vi "Simple ReaderWriteri.vi"() -> ()   [LabVIEW 2012]
uses:
  <vilib>/Platform/TimedLoop/XDataNode/timing_clust.ctl
  <vilib>/Platform/TimedLoop/XDataNode/nitl_modes.ctl
  <vilib>/Platform/TimedLoop/XDataNode/wakeup.ctl
  <vilib>/rvi/Emulation/niFpgaSctlEmulationRegisterWithScheduler.vi
  <vilib>/rvi/eio/common/nirviEmuTemplateMethod_errors.vi
  <vilib>/rvi/Emulation/niFpgaSctlEmulationScheduler.vi
  <vilib>/rvi/interface/RandomDataEmulation/nirviRandomDataFPGAFIFO.vi
  <vilib>/rvi/interface/RandomDataEmulation/niFpgaRandomDataHandleErrors.vi
  <vilib>/Platform/TimedLoop/XDataNode/XDataNode.xnode
  <vilib>/eio/EIONode/EIONode.xnode
  <vilib>/rvi/DataTransferAndStorage/Container/XNode/niFpgaContainer.xnode
  <vilib>/rvi/interface/RandomDataEmulation/nirviRandomDataFpgaReadWriteTemplate.vi
  <vilib>/Platform/TimedLoop/XDataNode/XDNodeRunTimeDep.lvlib
panel:
  out "All samples acquired":bool
  in  "Write array (Ch1)":bool[](array[boolean])=[FALSE, FALSE, FALSE, FALSE, FALSE, FALSE, FALSE, FALSE, FALSE, FALSE, FALSE, FALSE, FALSE, FALSE, FALSE, FALSE]
  in  "Samples":i32
  in  "Onboard_Clock_Write_Data":u16 format="%b"
  in  "Onboard_Clock_Write":bool
  out "Onboard_Clock_Ready":bool
  out "Read array (Ch0)":bool[](array[boolean])
  in  "Acq_Reset":bool
  in  "Clock Source":u8(ring)=3 items=["Tristate"=0, "Sync Clock (PXIe Only)"=2, "Adapter Module Onboard Clock"=3, "Strobe From Crosspoint Switch"=4, "Strobe Bypass"=5]
  in  "Xpoint_Switch_Write":bool
  out "Xpoint_Switch_Ready":bool
  in  "Commit":bool
  # "Configuration"
  # "Read on Ch0, Write on Ch1"
  # "Generation"
  # "Acquisition"
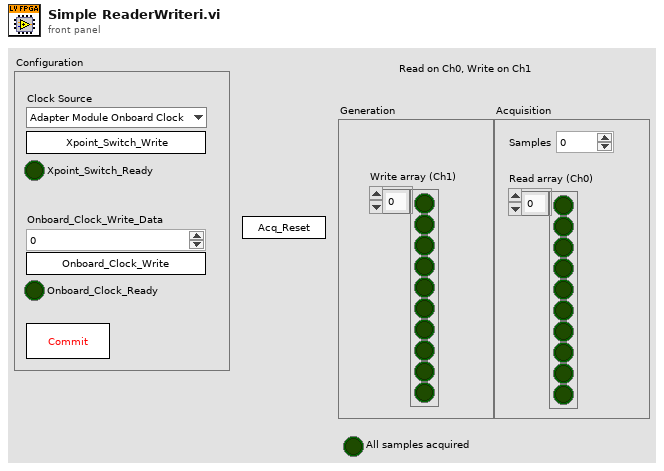
[diagram p1: front panel]
types:
  T1 = typedef "XDNodeRunTimeDep.lvlib/timing_clust.ctl" = cluster{"Expected End [f-1]":u64, "Actual End [f-1]":u64, "Finished Late? [f-1]":bool, "Expected End [i-1]":u64, "Actual End [i-1]":u64, "Finished Late? [i-1]":bool, "Expected Start [i]":u64, "Actual Start [i]":u64, "Expected Start [f]":u64, "Actual Start [f]":u64, "Source Name":string, "Structure Name":string, "Period":i64, "Deadline":i64, "Offset":i64, "Start":i64, "Priority":i32, "Timeout":i32, "Mode":T2, "Wakeup Reason":T3, "Error":errorcluster, "Source Type":string, "Secondary Source Type":string, "Global End Time":u64, "Global Start Time":u64, "Frame Duration":u64, "Iteration Duration":u64, "Assigned CPU":i32, "I/O Scan Engine Mode":u32}
  T2 = typedef "XDNodeRunTimeDep.lvlib/nitl_modes.ctl" = enum32{"No Change", "Process missed periods, maintain original phase", "Discard missed periods, maintain original phase", "Process missed periods, ignore original phase", "Discard missed periods, ignore original phase"}
  T3 = typedef "XDNodeRunTimeDep.lvlib/wakeup.ctl" = enum32{"Normal", "Aborted", "Asynchronous wakeup", "Timing source error", "Timed loop error", "Timeout"}
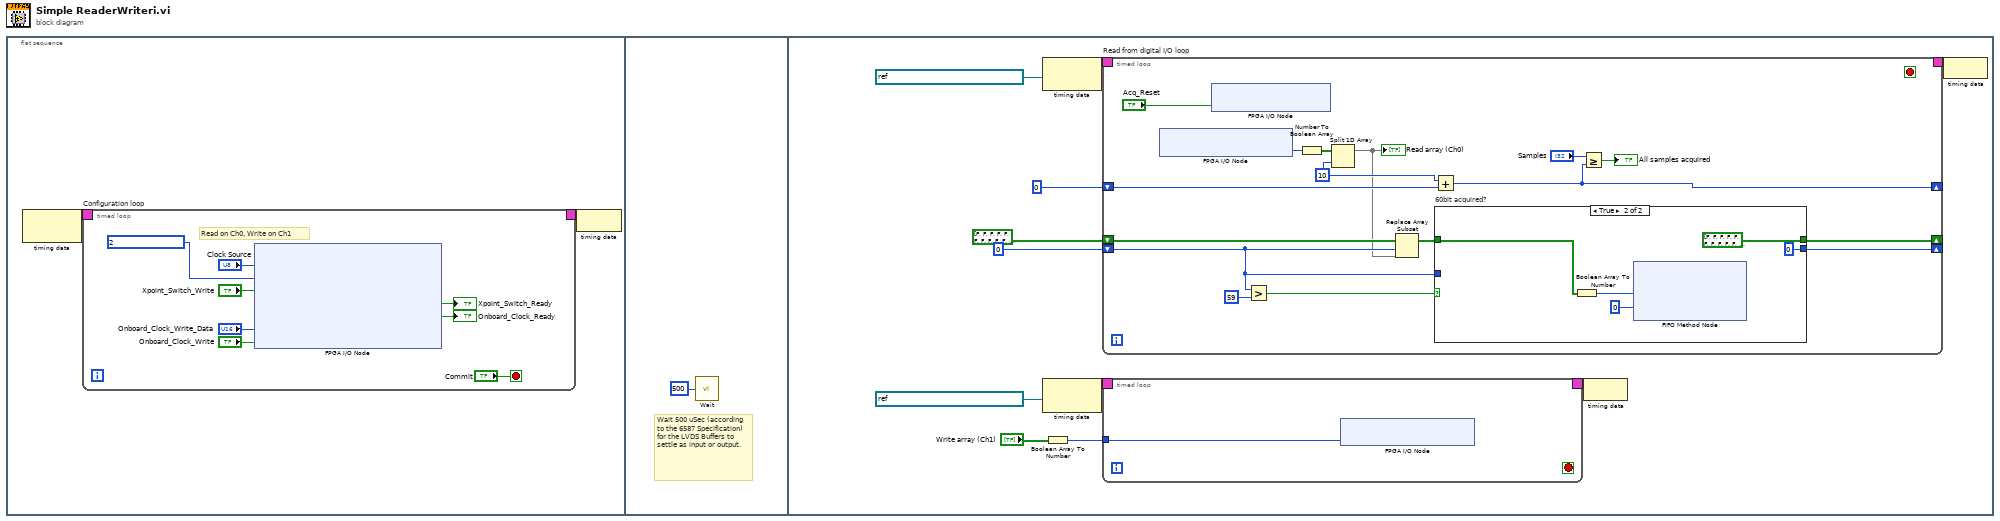
[diagram p0: block diagram]
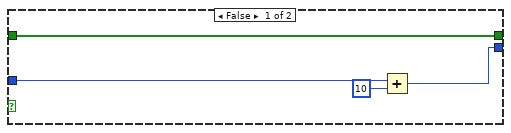
[diagram p2: hidden frame]
diagram:
  n1 = flat-sequence {
    frame #0 {
      n2 = node-c288() -> (w2:T1)  [unwired: 1 in]
      n3 = timed-loop "Configuration loop" {
        timing: w2 -> [_]
        timing-out: [_] -> w1
        stop <- "Commit" stop-if-true
        # "Read on Ch0, Write on Ch1"
        n4 = xnode "FPGA I/O Node"("IO Module\\Acq_IO_Clock_Source"="Clock Source", "IO Module\\LVDS_Data_Dir"=u16 2 ("IO Module\\LVDS_Data_Dir"), "IO Module\\Xpoint_Switch_Write"="Xpoint_Switch_Write", "IO Module\\Onboard_Clock_Write_Data"="Onboard_Clock_Write_Data", "IO Module\\Onboard_Clock_Write"="Onboard_Clock_Write") -> ("IO Module\\Xpoint_Switch_Ready"=→"Xpoint_Switch_Ready":bool, "IO Module\\Onboard_Clock_Ready"=→"Onboard_Clock_Ready":bool)  [unwired: 7 in, 7 out]
      }
      n5 = node-c288(w1) -> ()
    }
    frame #1 {
      # "Wait 500 uSec (according to the 6587 Specification) for the LVDS Buffers to settle as input or output."
      n6 = call "Wait"("Count(uSec)"=u32 500) -> ()  [unwired: 1 out]
    }
    frame #2 {
      n7 = node-c288(refnum<k21> "IO Module\\Acq_Regional_Clock" ("Source Name")) -> (w26:T1)
      n8 = node-c288(refnum<k21> "IO Module\\Gen_Regional_Clock" ("Source Name")) -> (w20:T1)
      n9 = Boolean Array To Number(Boolean array="Write array (Ch1)") -> (number=w16:u16)
      n10 = timed-loop "Read from digital I/O loop" {
        timing: w26 -> [_]
        timing-out: [_] -> w25
        shift-right: [w44] -> _
        shift-left: 0 -> [w37]
        shift-right: [w45] -> _
        shift-left: bool[] [FALSE, FALSE, FALSE, FALSE, FALSE, FALSE, FALSE, FALSE, FALSE, FALSE, FALSE, FALSE, FALSE, FALSE, FALSE, FALSE, FALSE, FALSE, FALSE, FALSE, FALSE, FALSE, FALSE, FALSE, FALSE, FALSE, FALSE, FALSE, FALSE, FALSE, FALSE, FALSE, FALSE, FALSE, FALSE, FALSE, FALSE, FALSE, FALSE, FALSE, FALSE, FALSE, FALSE, FALSE, FALSE, FALSE, FALSE, FALSE, FALSE, FALSE, FALSE, FALSE, FALSE, FALSE, FALSE, FALSE, FALSE, FALSE, FALSE, FALSE, FALSE, FALSE, FALSE, FALSE] ("Boolean array") -> [w38]
        shift-right: [w41] -> _
        shift-left: 0 -> [w43]
        stop <- _ stop-if-true
        w42 = 10 ("index")
        n11 = xnode "FPGA I/O Node"() -> ("IO Module\\LVDS_Ch0_Rd"=w48:u16)  [unwired: 1 in, 1 out]
        n12 = xnode "FPGA I/O Node"("IO Module\\Acq_Reset"="Acq_Reset") -> ()  [unwired: 1 in, 1 out]
        n13 = Greater?(x=w37, y=59) -> (0:w39:bool)
        n14 = Number To Boolean Array(number=w48) -> (Boolean array=w47:bool[])
        n15 = Split 1D Array(array=w47, index=w42) -> (first subarray=w36:bool[])  [unwired: 1 out]
        "Read array (Ch0)" <- w36
        n16 = Replace Array Subset(array=w38, new element=w36, index=w37) -> (w35:bool[])
        n17 = Add(x=w42, y=w43) -> (x+y=w41:i32)
        n18 = case "60bit acquired?" shown="True" w39 {
          tunnel: [w50 bool[] [FALSE, FALSE, FALSE, FALSE, FALSE, FALSE, FALSE, FALSE, FALSE, FALSE, FALSE, FALSE, FALSE, FALSE, FALSE, FALSE, FALSE, FALSE, FALSE, FALSE, FALSE, FALSE, FALSE, FALSE, FALSE, FALSE, FALSE, FALSE, FALSE, FALSE, FALSE, FALSE, FALSE, FALSE, FALSE, FALSE, FALSE, FALSE, FALSE, FALSE, FALSE, FALSE, FALSE, FALSE, FALSE, FALSE, FALSE, FALSE, FALSE, FALSE, FALSE, FALSE, FALSE, FALSE, FALSE, FALSE, FALSE, FALSE, FALSE, FALSE, FALSE, FALSE, FALSE, FALSE] ("Boolean array")] -> w45
          tunnel: [w52 0] -> w44
          tunnel: w37 -> [w53 _]
          tunnel: w35 -> [w50 w54]
          frame False {
            n19 = Add(x=w53, y=10) -> (x+y=w52:i32)
          }
          frame True {
            n20 = Boolean Array To Number(Boolean array=w54) -> (number=w58:u64)
            n21 = xnode ("FIFO Method Node")("Element"=w58, "Timeout"=0) -> ()  [unwired: 1 in, 2 out]
          }
        }
        n22 = Greater Or Equal?(x="Samples", y=w41) -> (x >= y?=→"All samples acquired":bool)
      }
      n23 = timed-loop {
        timing: w20 -> [_]
        timing-out: [_] -> w19
        tunnel: w16 -> [w27]
        stop <- _ stop-if-true
        n24 = xnode "FPGA I/O Node"("IO Module\\LVDS_Ch1_Wr"=w27) -> ()  [unwired: 1 in, 1 out]
      }
      n25 = node-c288(w19) -> ()
      n26 = node-c288(w25) -> ()
    }
  }
